vi "UpdateParams.vi"(11 "FPGA in":refnum<queue>) -> (3 "FPGA out":refnum<queue>)   [LabVIEW 2019, in "FPGA.lvlib"]
uses:
  FPGA.lvlib
  FPGA.ctl
panel:
  out "FPGA CLUSTER":T1={"Start freq. [Hz]"=10.0, "Sweep duration [s]"=0.1, "Freq. step [Hz]"=0.1, "DAC Sample Rate"=1388888.8888, "ADC Sample Rate"=50000000.0, "CMD port"=2047, "DFAST port"=2048, "CMD ID"=refnum, "DFAST ID"=refnum, "CMD error out"={"status"=FALSE, "code"=0, "source"=""}, "FPGA IP"="192.168.1.12", "DFAST error out "={"status"=FALSE, "code"=0, "source"=""}, "Stop freq. [Hz]"=0.0, "Discrete sweep"=FALSE, "Initial NCO"=10, "Difference NCO"=0, "step NCO"=0, "Final NCO"=0, "clocks for step"=0, "demodulation"=FALSE, "NCO Phase Precision"=32, "NCO Sample Rate"=50000000.0, "Time for step [s]"=0.1, "NCO freq. resolution"=32.0, "Sweep speed [Hz/s]"=0.1, "Connected"=FALSE, "Slew Rate [V/us]"=0.8, "Parameters_ok"=FALSE, "Amplitude [mVpp]"=10.0, "Scale Factor"=0.999969482421875, "Acquiring"=FALSE, "DAC-ADC Latency"=1, "Digital Gain"=0, "Number of steps"=1, "Averaging preferred"=FALSE, "Filter Order"=1, "Settling"=enum."99,9%"} {"Filter Order" min=1 max=4; "Number of steps" min=1; "Digital Gain" items=["1", "2", "4", "8", "16", "32", "64"]; "DAC-ADC Latency" min=1 format="%#_4g"; "Scale Factor" format="%#_4g"; "Amplitude [mVpp]" min=4.0 max=200.0 format="%.3f"; "Sweep speed [Hz/s]" min=0.001 max=5.0 step=0.001 format="%.3f"; "Time for step [s]" min=0.001 max=5.0 step=0.001 format="%.3f"; "clocks for step" min=1 max=5 step=1; "Final NCO" min=4 max=200; "step NCO" min=1 max=5 step=1; "Difference NCO" min=1 max=5 step=1; "Initial NCO" min=4 max=200; "Stop freq. [Hz]" min=4.0 max=200.0 format="%.3f"; "Freq. step [Hz]" min=0.001 max=5.0 step=0.001 format="%.3f"; "Sweep duration [s]" min=0.001 max=5.0 step=0.001 format="%.3f"; "Start freq. [Hz]" min=4.0 max=200.0 format="%.3f"}
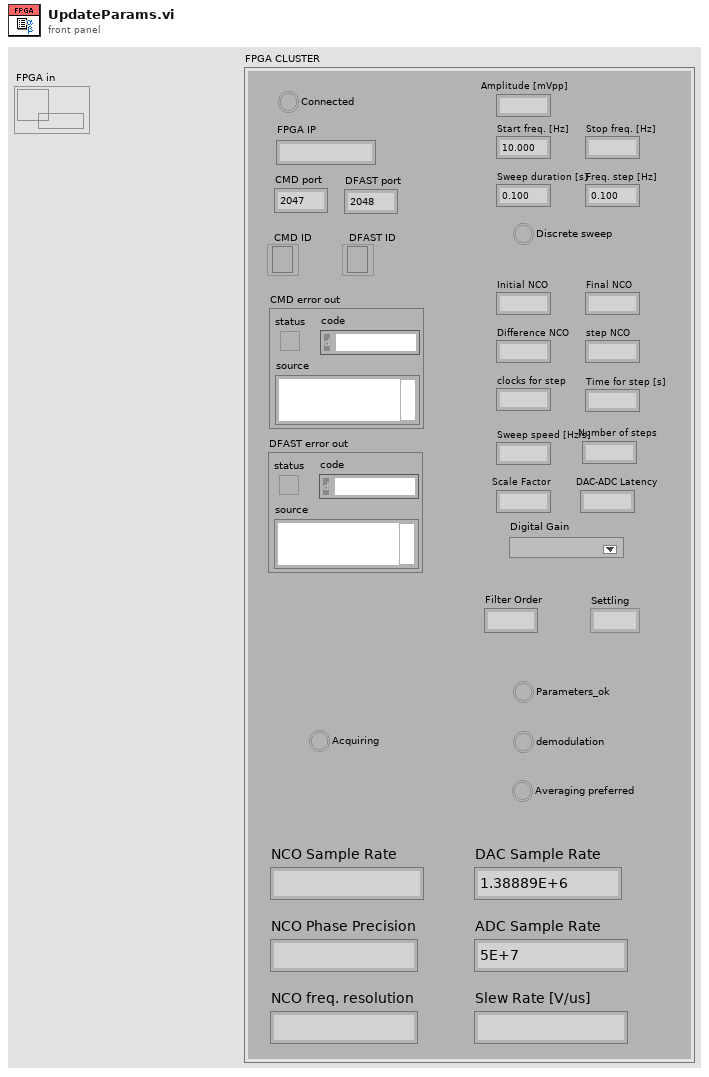
[diagram p1: front panel]
types:
  T1 = typedef "FPGA.lvlib/FPGA.ctl" = cluster{"Start freq. [Hz]":dbl, "Sweep duration [s]":dbl, "Freq. step [Hz]":dbl, "DAC Sample Rate":dbl, "ADC Sample Rate":dbl, "CMD port":u16, "DFAST port":u16, "CMD ID":refnum<k16>, "DFAST ID":refnum<k16>, "CMD error out":errorcluster, "FPGA IP":string, "DFAST error out ":errorcluster, "Stop freq. [Hz]":dbl, "Discrete sweep":bool, "Initial NCO":u32, "Difference NCO":i32, "step NCO":i64, "Final NCO":u32, "clocks for step":u32, "demodulation":bool, "NCO Phase Precision":u32, "NCO Sample Rate":dbl, "Time for step [s]":dbl, "NCO freq. resolution":dbl, "Sweep speed [Hz/s]":dbl, "Connected":bool, "Slew Rate [V/us]":dbl, "Parameters_ok":bool, "Amplitude [mVpp]":dbl, "Scale Factor":fxp<+,16,0>, "Acquiring":bool, "DAC-ADC Latency":u16, "Digital Gain":i32, "Number of steps":i32, "Averaging preferred":bool, "Filter Order":u32, "Settling":enum16{"99%", "99,9%"}}
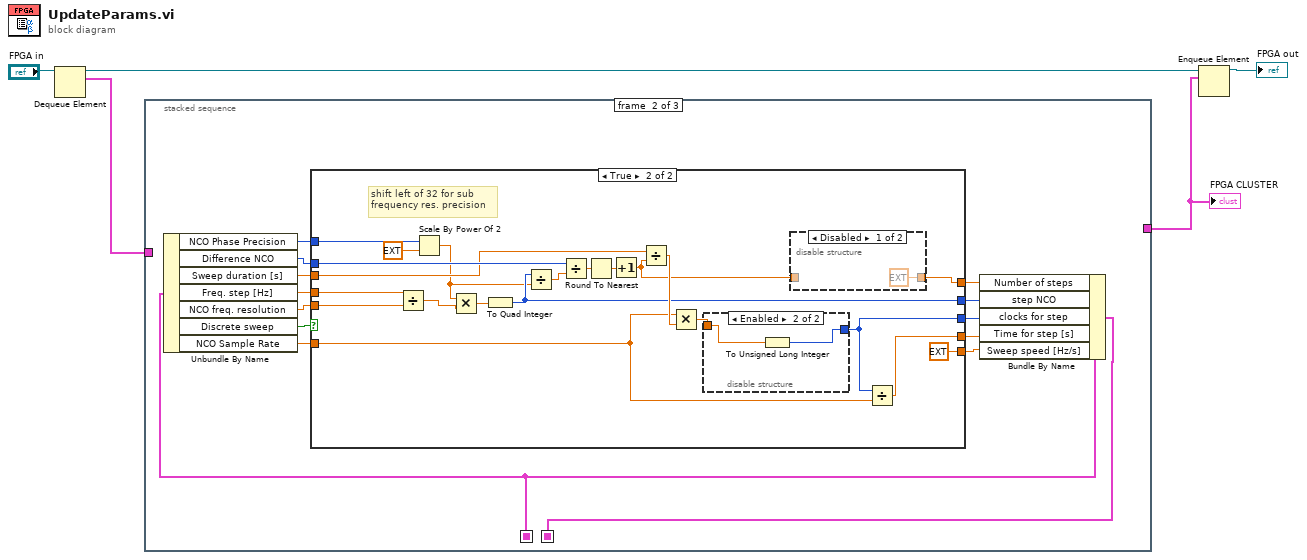
[diagram p0: block diagram]
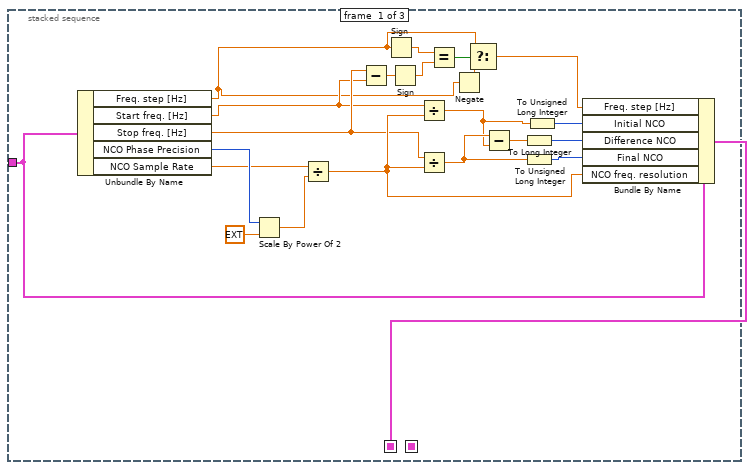
[diagram p2: hidden frame]
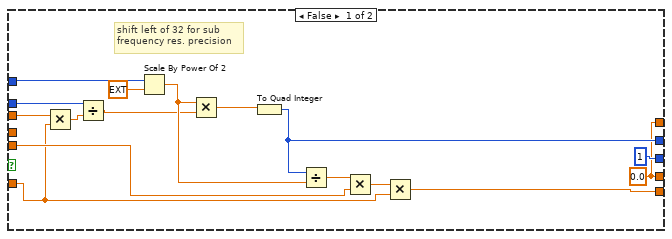
[diagram p3: hidden frame]
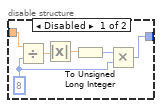
[diagram p5: hidden frame]
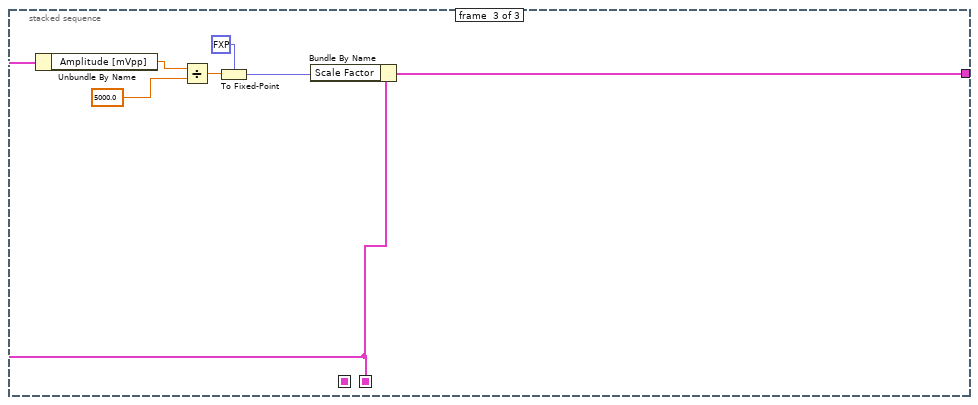
[diagram p6: hidden frame]
diagram:
  n1 = Dequeue Element(queue="FPGA in") -> (queue out=w4:refnum<queue>, element=w2:T1)  [unwired: 2 in, 2 out]
  n2 = stacked-sequence {
    seq-local: [w19 _ _] -> [_ w41 _]
    seq-local: [_ w29 _] -> [_ _ w90]
    tunnel: w2 -> [w15 _ _]
    tunnel: [_ _ w89] -> w1
    frame #0 {
      n3 = Unbundle By Name(w15) -> ("Freq. step [Hz]"=w7:dbl, "Start freq. [Hz]"=w13:dbl, "Stop freq. [Hz]"=w14:dbl, "NCO Phase Precision"=w26:u32, "NCO Sample Rate"=w16:dbl)
      n4 = Scale By Power Of 2(n=w26, x=ext 1.0) -> (x*2^n=w17:ext)
      n5 = Divide(x=w16, y=w17) -> (x/y=w18:ext)
      n6 = Subtract(x=w14, y=w13) -> (x-y=w12:dbl)
      n7 = Sign(1:w7) -> (0:w11:dbl)
      n8 = Sign(1:w12) -> (0:w10:dbl)
      n9 = Divide(x=w13, y=w18) -> (x/y=w22:ext)
      n10 = Divide(x=w14, y=w18) -> (x/y=w24:ext)
      n11 = Equal?(x=w11, y=w10) -> (x = y?=w9:bool)
      n12 = Negate(x=w7) -> (-x=w8:dbl)
      n13 = Select(t=w7, s=w9, f=w8) -> (s? t:f=w6:dbl)
      n14 = Subtract(x=w24, y=w22) -> (x-y=w25:ext)
      n15 = To Long Integer(number=w25) -> (32bit integer=w20:i32)
      n16 = To Unsigned Long Integer(number=w24) -> (unsigned 32bit integer=w23:u32)
      n17 = To Unsigned Long Integer(number=w22) -> (unsigned 32bit integer=w21:u32)
      n18 = Bundle By Name(cluster=w15, "Freq. step [Hz]"=w6, "Initial NCO"=w21, "Difference NCO"=w20, "Final NCO"=w23, "NCO freq. resolution"=w18) -> (w19:T1)
    }
    frame #1 {
      n19 = Unbundle By Name(w41) -> ("NCO Phase Precision"=w31:u32, "Difference NCO"=w36:i32, "Sweep duration [s]"=w35:dbl, "Freq. step [Hz]"=w39:dbl, "NCO freq. resolution"=w38:dbl, "Discrete sweep"=w40:bool, "NCO Sample Rate"=w34:dbl)
      n20 = case shown="True" w40 {
        tunnel: w39 -> [_ w78]
        tunnel: w38 -> [w49 w77]
        tunnel: [w52 w71] -> w37
        tunnel: w36 -> [w56 w76]
        tunnel: w35 -> [w45 w75]
        tunnel: w34 -> [w44 w73]
        tunnel: [u32 1 w62] -> w33
        tunnel: [w42 w72] -> w32
        tunnel: w31 -> [w54 w70]
        tunnel: [w47 ext 0.0] -> w30
        tunnel: [w42 w59] -> w28
        frame False {
          w42 = 0.0
          # "shift left of 32 for sub\nfrequency res. precision"
          n21 = Multiply(x=w45, y=w44) -> (x*y=w46:dbl)
          n22 = Divide(x=w56, y=w46) -> (x/y=w43:dbl)
          n23 = Scale By Power Of 2(n=w54, x=ext 1.0) -> (x*2^n=w51:ext)
          n24 = Multiply(x=w51, y=w43) -> (x*y=w53:ext)
          n25 = To Quad Integer(1:w53) -> (0:w52:i64)
          n26 = Divide(x=w52, y=w51) -> (x/y=w50:ext)
          n27 = Multiply(x=w50, y=w49) -> (x*y=w48:ext)
          n28 = Multiply(x=w48, y=w44) -> (x*y=w47:ext)
        }
        frame True {
          # "shift left of 32 for sub\nfrequency res. precision"
          n29 = Divide(x=w78, y=w77) -> (x/y=w67:dbl)
          n30 = Scale By Power Of 2(n=w70, x=ext 1.0) -> (x*2^n=w68:ext)
          n31 = Multiply(x=w68, y=w67) -> (x*y=w66:ext)
          n32 = To Quad Integer(1:w66) -> (0:w71:i64)
          n33 = Divide(x=w71, y=w68) -> (x/y=w65:ext)
          n34 = Divide(x=w76, y=w65) -> (x/y=w61:ext)
          n35 = Round To Nearest(number=w61) -> (nearest integer value=w60:ext)
          n36 = Increment(x=w60) -> (x+1=w58:ext)
          n37 = Divide(x=w75, y=w58) -> (x/y=w74:ext)
          n38 = Multiply(x=w73, y=w74) -> (x*y=w63:ext)
          n39 = disable-structure shown="Enabled" {
            disable-tunnel: w63 -> [w86 w88]
            disable-tunnel: [w84 w87] -> w62
            frame Disabled {
              w81 = u32 8 ("y")
              n40 = Divide(x=w86, y=w81) -> (x/y=w83:ext)
              n41 = Absolute Value(x=w83) -> (abs(x)=w82:ext)
              n42 = To Unsigned Long Integer(number=w82) -> (unsigned 32bit integer=w85:u32)
              n43 = Multiply(x=w85, y=w81) -> (x*y=w84:u32)
            }
            frame Enabled {
              n44 = To Unsigned Long Integer(number=w88) -> (unsigned 32bit integer=w87:u32)
            }
          }
          n45 = disable-structure shown="Disabled" {
            disable-tunnel: [ext 1.0 w80] -> w59
            disable-tunnel: w58 -> [_ w80]
            frame Disabled {
            }
            frame Enabled {
            }
          }
          n46 = Divide(x=w62, y=w73) -> (x/y=w72:dbl)
        }
      }
      n47 = Bundle By Name(cluster=w41, "Number of steps"=w28, "step NCO"=w37, "clocks for step"=w33, "Time for step [s]"=w32, "Sweep speed [Hz/s]"=w30) -> (w29:T1)
    }
    frame #2 {
      n48 = Unbundle By Name(w90) -> ("Amplitude [mVpp]"=w95:dbl)
      n49 = Divide(x=w95, y=5000.0) -> (x/y=w91:dbl)
      n50 = To Fixed-Point(fixed-point type=fxp<+,16,0> 0.0 ("Numeric"), number=w91) -> (fixed-point=w92:fxp<+,16,0>)
      n51 = Bundle By Name(cluster=w90, "Scale Factor"=w92) -> (w89:T1)
    }
  }
  "FPGA CLUSTER" <- w1
  n52 = Enqueue Element(queue=w4, element=w1) -> (queue out=→"FPGA out":refnum<queue>)  [unwired: 2 in, 2 out]
